vi "VTI read all sensors.vi"(8 "error in (no error)":errorcluster, 11 "VISA Refnum in":refnum<visa-resource-name>) -> (0 "error out":errorcluster, 2 "TC sensors [K]":T1={"VTI space"=0.0, "Sample"=0.0, "He pot"=0.0, "Trap"=0.0, "Ambient"=0.0, "SetP_VTI"=0.0, "SetP_Smp"=0.0, "SetP_Pot"=0.0, "SetP_Trap"=0.0, "Range out 1"=1, "Out 1 [%]"=0.0, "Out 2 [%]"=0.0} {"Range out 1" items=["Off", "Range 1 (On)", "Range 2", "Range 3", "Range 4", "Range 5"]}, 3 "VISA Refnum out":refnum<visa-resource-name>)   [LabVIEW 2021, in "Temperature controller.lvlib"]
uses:
  Temperature controller.lvlib
  ctl/TC sensors.ctl
  <instrlib>/Lake Shore 350/Public/Data/Sensor Data (Single Reading).vi
  <instrlib>/Lake Shore 350/Lake Shore 350.lvlib
panel:
  out "Manual Output (0.00 %)":dbl format="%.2f"
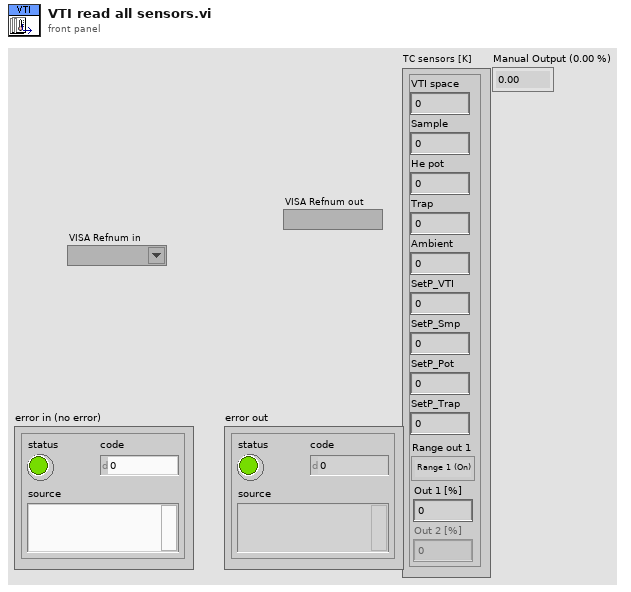
[diagram p1: front panel]
types:
  T1 = typedef "Temperature controller.lvlib/TC sensors.ctl" = cluster{"VTI space":dbl, "Sample":dbl, "He pot":dbl, "Trap":dbl, "Ambient":dbl, "SetP_VTI":dbl, "SetP_Smp":dbl, "SetP_Pot":dbl, "SetP_Trap":dbl, "Range out 1":u16, "Out 1 [%]":dbl, "Out 2 [%]":dbl}
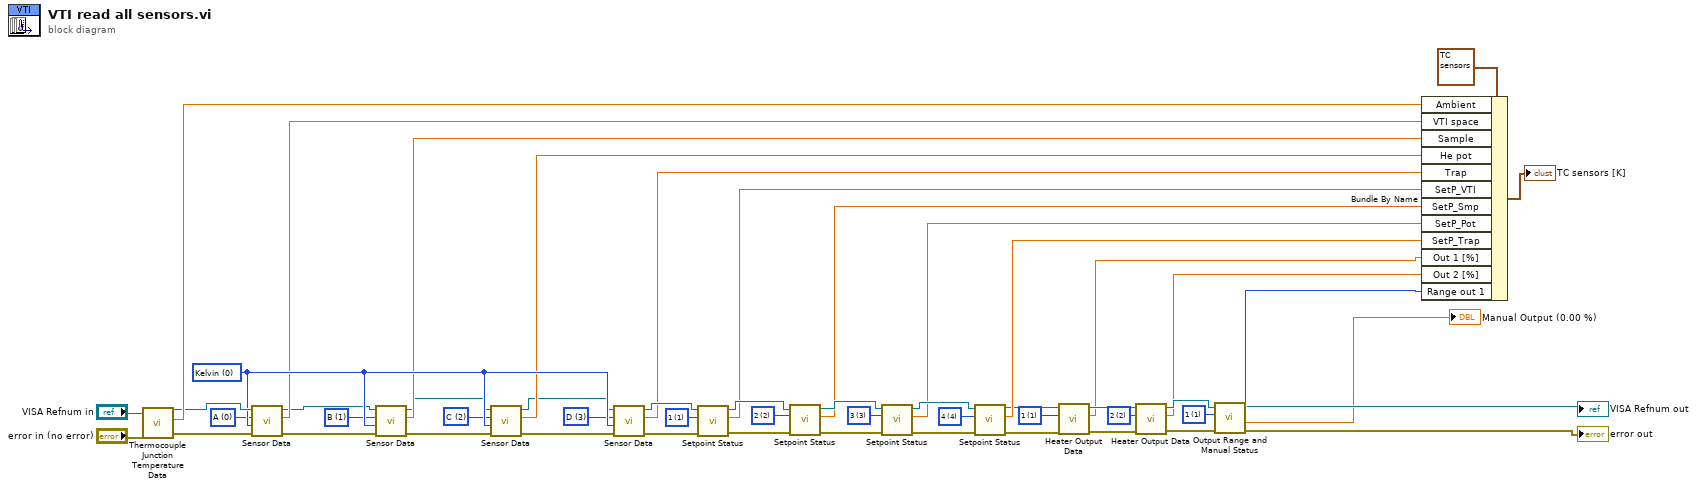
[diagram p0: block diagram]
diagram:
  w5 = u16 1 items=["1"=1, "2"=2, "3"=3, "4"=4] ("Output (1:1)")
  w8 = u16 2 items=["1"=1, "2"=2] ("Heater Output (1:1)")
  w11 = u16 1 items=["1"=1, "2"=2] ("Heater Output (1:1)")
  w22 = u16 4 items=["1"=1, "2"=2, "3"=3, "4"=4] ("Output (1:1)")
  w21 = u16 3 items=["1"=1, "2"=2, "3"=3, "4"=4] ("Output (1:1)")
  w23 = u16 2 items=["1"=1, "2"=2, "3"=3, "4"=4] ("Output (1:1)")
  w24 = u16 1 items=["1"=1, "2"=2, "3"=3, "4"=4] ("Output (1:1)")
  w48 = u16 0 items=["Kelvin", "Celsius", "Sensor Units"] ("Data Source (0:Kelvin)")
  w35 = u16 3 items=["A", "B", "C", "D", "D2", "D3", "D4", "D5"] ("Input (0:A)")
  w36 = u16 2 items=["A", "B", "C", "D", "D2", "D3", "D4", "D5"] ("Input (0:A)")
  w37 = u16 1 items=["A", "B", "C", "D", "D2", "D3", "D4", "D5"] ("Input (0:A)")
  w34 = u16 0 items=["A", "B", "C", "D", "D2", "D3", "D4", "D5"] ("Input (0:A)")
  n1 = call <instrlib>:"Thermocouple Junction Temperature Data.vi"("error in (no error)"="error in (no error)", "VISA resource name"="VISA Refnum in") -> ("error out"=w50:errorcluster, "Room-Temperature Sensor Data"=w51:dbl, "VISA resource name out"=w49:refnum<visa-resource-name>)  [unwired: 7 in]
  n2 = call-poly <instrlib>:"Sensor Data.vi"("error in (no error)"=w50, "Data Source (0:Kelvin)"=w48, "Input (0:A)"=w34, "VISA resource name"=w49) -> ("error out"=w43:errorcluster, "Sensor Data"=w47:dbl, "VISA resource name out"=w38:refnum<visa-resource-name>)  [unwired: 5 in]
  n3 = call-poly <instrlib>:"Sensor Data.vi"("error in (no error)"=w43, "Data Source (0:Kelvin)"=w48, "Input (0:A)"=w37, "VISA resource name"=w38) -> ("error out"=w42:errorcluster, "Sensor Data"=w46:dbl, "VISA resource name out"=w39:refnum<visa-resource-name>)  [unwired: 5 in]
  n4 = call-poly <instrlib>:"Sensor Data.vi"("error in (no error)"=w42, "Data Source (0:Kelvin)"=w48, "Input (0:A)"=w36, "VISA resource name"=w39) -> ("error out"=w41:errorcluster, "Sensor Data"=w45:dbl, "VISA resource name out"=w40:refnum<visa-resource-name>)  [unwired: 5 in]
  n5 = call-poly <instrlib>:"Sensor Data.vi"("error in (no error)"=w41, "Data Source (0:Kelvin)"=w48, "Input (0:A)"=w35, "VISA resource name"=w40) -> ("error out"=w20:errorcluster, "Sensor Data"=w44:dbl, "VISA resource name out"=w52:refnum<visa-resource-name>)  [unwired: 5 in]
  n6 = call <instrlib>:"Setpoint Status.vi"("error in (no error)"=w20, "Output (1:1)"=w24, "VISA resource name"=w52) -> ("error out"=w25:errorcluster, "Setpoint"=w16:dbl, "VISA resource name out"=w26:refnum<visa-resource-name>)  [unwired: 6 in]
  n7 = call <instrlib>:"Setpoint Status.vi"("error in (no error)"=w25, "Output (1:1)"=w23, "VISA resource name"=w26) -> ("error out"=w30:errorcluster, "Setpoint"=w19:dbl, "VISA resource name out"=w29:refnum<visa-resource-name>)  [unwired: 6 in]
  n8 = call <instrlib>:"Setpoint Status.vi"("error in (no error)"=w30, "Output (1:1)"=w21, "VISA resource name"=w29) -> ("error out"=w28:errorcluster, "Setpoint"=w18:dbl, "VISA resource name out"=w27:refnum<visa-resource-name>)  [unwired: 6 in]
  n9 = call <instrlib>:"Setpoint Status.vi"("error in (no error)"=w28, "Output (1:1)"=w22, "VISA resource name"=w27) -> ("error out"=w13:errorcluster, "Setpoint"=w17:dbl, "VISA resource name out"=w12:refnum<visa-resource-name>)  [unwired: 6 in]
  n10 = call <instrlib>:"Heater Output Data.vi"("error in (no error)"=w13, "Heater Output (1:1)"=w11, "VISA resource name"=w12) -> ("error out"=w15:errorcluster, "Output Value"=w7:dbl, "VISA resource name out"=w14:refnum<visa-resource-name>)  [unwired: 6 in]
  n11 = call <instrlib>:"Heater Output Data.vi"("error in (no error)"=w15, "Heater Output (1:1)"=w8, "VISA resource name"=w14) -> ("error out"=w10:errorcluster, "Output Value"=w6:dbl, "VISA resource name out"=w9:refnum<visa-resource-name>)  [unwired: 6 in]
  n12 = call <instrlib>:"Output Range and Manual Status.vi"("error in (no error)"=w10, "Output (1:1)"=w5, "VISA resource name"=w9) -> ("error out"=→"error out":errorcluster, "Manual Output (0.00 %)"=→"Manual Output (0.00 %)":dbl, "Range (0:Off)"=w4:u16, "VISA resource name out"=→"VISA Refnum out":refnum<visa-resource-name>)  [unwired: 5 in]
  n13 = Bundle By Name(cluster=T1 {"VTI space"=0.0, "Sample"=0.0, "He pot"=0.0, "Trap"=0.0, "Ambient"=0.0, "SetP_VTI"=0.0, "SetP_Smp"=0.0, "SetP_Pot"=0.0, "SetP_Trap"=0.0, "Range out 1"=1, "Out 1 [%]"=0.0, "Out 2 [%]"=0.0}, "Ambient"=w51, "VTI space"=w47, "Sample"=w46, "He pot"=w45, "Trap"=w44, "SetP_VTI"=w16, "SetP_Smp"=w19, "SetP_Pot"=w18, "SetP_Trap"=w17, "Out 1 [%]"=w7, "Out 2 [%]"=w6, "Range out 1"=w4) -> (→"TC sensors [K]":T1)
